vi "GetWaveformInfoArray.vi"(8 "error in (no error)":errorcluster, 11 "TektronixDPOSimple in":refnum<class "TektronixDPOSimple.lvclass">) -> (0 "error out":errorcluster, 3 "TektronixDPOSimple out":refnum<class "TektronixDPOSimple.lvclass">)   [LabVIEW 2020, in "TektronixDPOSimple.lvclass"]
doc: "Read the Waveform Info from the physical device"
uses:
  TektronixDPOSimple.lvclass
  TektronixDPOSimple.lvclass/TektronixDPOSimple.ctl
  Tektronix DPO MSO 2000 4000 Series.lvlib
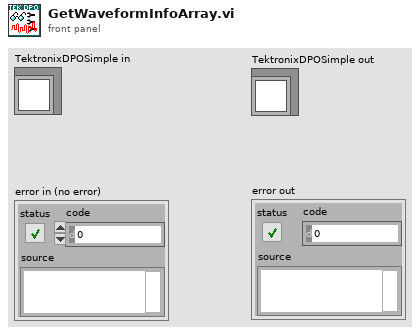
[diagram p1: front panel]
types:
  T1 = typedef "Waveform_attributes.ctl" = cluster{"t0":dbl, "dt":dbl, "multipler":dbl, "offset1":dbl, "offset2":dbl}
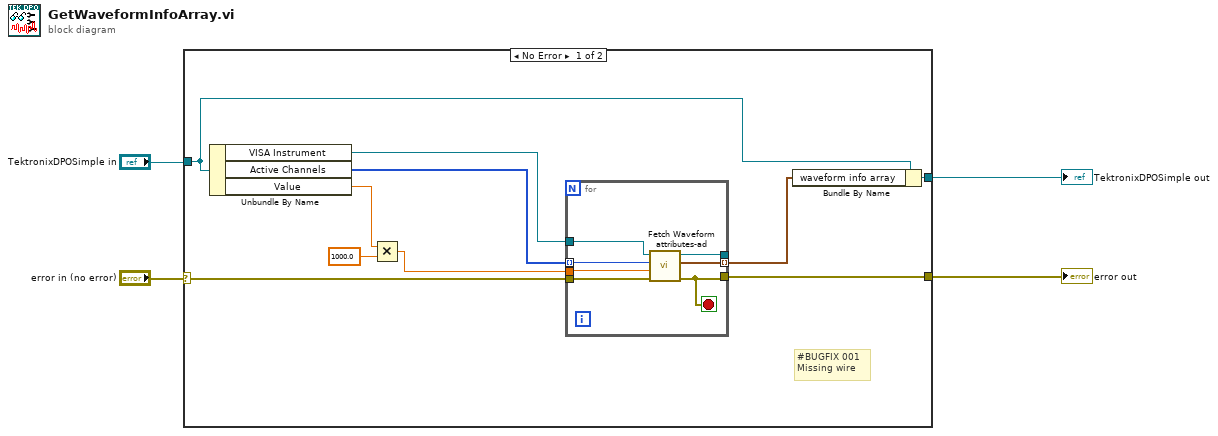
[diagram p0: block diagram]
diagram:
  n1 = case shown="No Error" "error in (no error)" {
    selector: "error in (no error)" -> [w11 w23]
    tunnel: "TektronixDPOSimple in" -> [w10 w22]
    tunnel: [w12 w23] -> w3
    tunnel: [w9 w22] -> w1
    frame No Error {
      # "#BUGFIX 001\nMissing wire"
      n2 = Unbundle By Name(w10) -> ("VISA Instrument"=w14:refnum<visa-resource-name>, "Active Channels"=w13:u16[], "Value"=w7:dbl)
      n3 = Multiply(x=w7, y=1000.0) -> (x*y=w5:dbl)
      n4 = for {
        tunnel: w14 -> [w21]
        tunnel: w13 -> [w20] mode=indexing
        tunnel: w11 -> [w19]
        tunnel: [w18] -> w12
        tunnel: [w17] -> _
        tunnel: [w16] -> w8 mode=indexing
        tunnel: w5 -> [w15]
        stop <- w18 stop-if-true
        n5 = call "Fetch Waveform attributes-ad.vi"("error in (no error)"=w19, "General Settings:Timeout Value"=w15, "Channel (0: Channel 1)"=w20, "VISA resource name"=w21) -> ("error out"=w18:errorcluster, "output cluster"=w16:T1, "VISA resource name out"=w17:refnum<visa-resource-name>)  [unwired: 5 in]
      }
      n6 = Bundle By Name(cluster=w10, "waveform info array"=w8) -> (w9:refnum<class "TektronixDPOSimple.lvclass">)
    }
    frame Error {
    }
  }
  "error out" <- w3
  "TektronixDPOSimple out" <- w1
